vi "Player Info.vi"(11 "Spread in":refnum<class "Spread.lvclass">) -> (1 "Victory Speech":string, 2 "Name":string, 3 "Spread out":refnum<class "Spread.lvclass">)   [LabVIEW 2015, in "Spread.lvclass"]
uses:
  Spread.lvclass
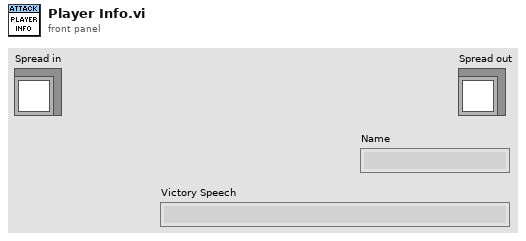
[diagram p1: front panel]
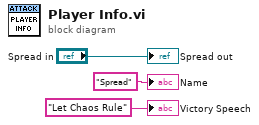
[diagram p0: block diagram]
diagram:
  "Spread out" <- "Spread in"
  "Name" <- "Spread" ("Name")
  "Victory Speech" <- "Let Chaos Rule" ("Victory Speech")
